vi "ADC_DAC_Trigger.vi"() -> ()   [LabVIEW 2018]
doc: "The DtAinContinuous example demonstrates how to continuously acquire data from an analog input channel. This example runs continuously until either the Stop button is pressed or an error occurs."
uses:
  <userlib>/LV-Link3/PolySubVIs/DtCreateAinChan.vi
  <userlib>/LV-Link3/PolySubVIs/DtOLWriteMultiple2D.vi
  <userlib>/LV-Link3/PolySubVIs/DtOLTimingSetInput.vi
  <vilib>/Waveform/WDTFileIO.llb/Export Waveform To Spreadsheet File.vi
  <vilib>/Analysis/baseanly.llb/Mean (DBL).vi
  <vilib>/Analysis/NI_AALBase.lvlib
  <vilib>/measure/mamon.llb/Trigger Detection for 1 Channel.vi
  <vilib>/measure/NI_MAPro.lvlib
  <userlib>/LV-Link3/PolySubVIs/DtCreateAoutChan.vi
panel:
  in  "Tab Control":T1(tab)
  in  "Device":string(combo)="DT9816-S(00)"
  in  "Device 2":string(combo)="DT9854(00)"
  in  "ADC Channels":string="0, 1, 2, 3, 4"
  in  "Sample Rate":u32=10000
  in  "Samples Per Channel":i32=1000
  in  "Sync Mode":i32(ring) items=["None", "Master", "Slave"]
  in  "Start Button":bool
  in  "Stop Button":bool
  in  "DAC Channels":string="0, 1, 2, 3, 4"
  in  "?":bool
  in  "Trigger Channel":i8 min=0 max=5
  in  "location mode":u16(ring) items=["Index", "Time"]
  in  "trigger slope":u16(ring)=1 items=["Falling Edge", "Rising Edge"]
  in  "DAC Channel 0":dbl=0.22199999999999995 min=0.0 max=1.125 step=0.01
  in  "DAC Channel 1":dbl=0.5200000000000001 min=0.0 max=1.125 step=0.01
  in  "DAC Channel 2":dbl=0.42000000000000015 min=0.0 max=1.125 step=0.01
  in  "DAC Channel 3":dbl=0.41000000000000014 min=0.0 max=1.125 step=0.01
  in  "DAC Channel 4":dbl=0.5200000000000001 min=0.0 max=1.125 step=0.01
  out "Signal from two channel":dbl[][](graph)
  out "Signal from two channel":dbl[][](graph)
  out "Waveform Chart":dbl(graph)
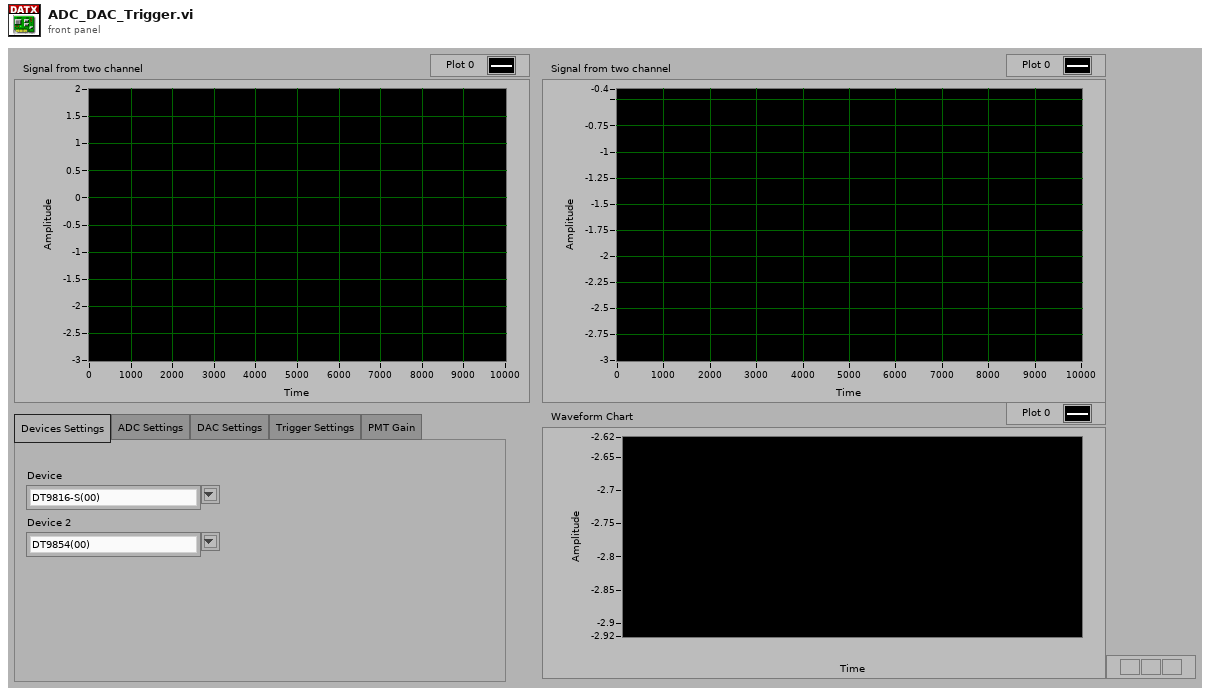
[diagram p1: front panel]
types:
  T1 = enum32{"Devices Settings", "ADC Settings", "DAC Settings", "Trigger Settings", "PMT Gain"}
  T2 = enum8{"Enabled", "Disabled", "Disabled and Grayed Out"}
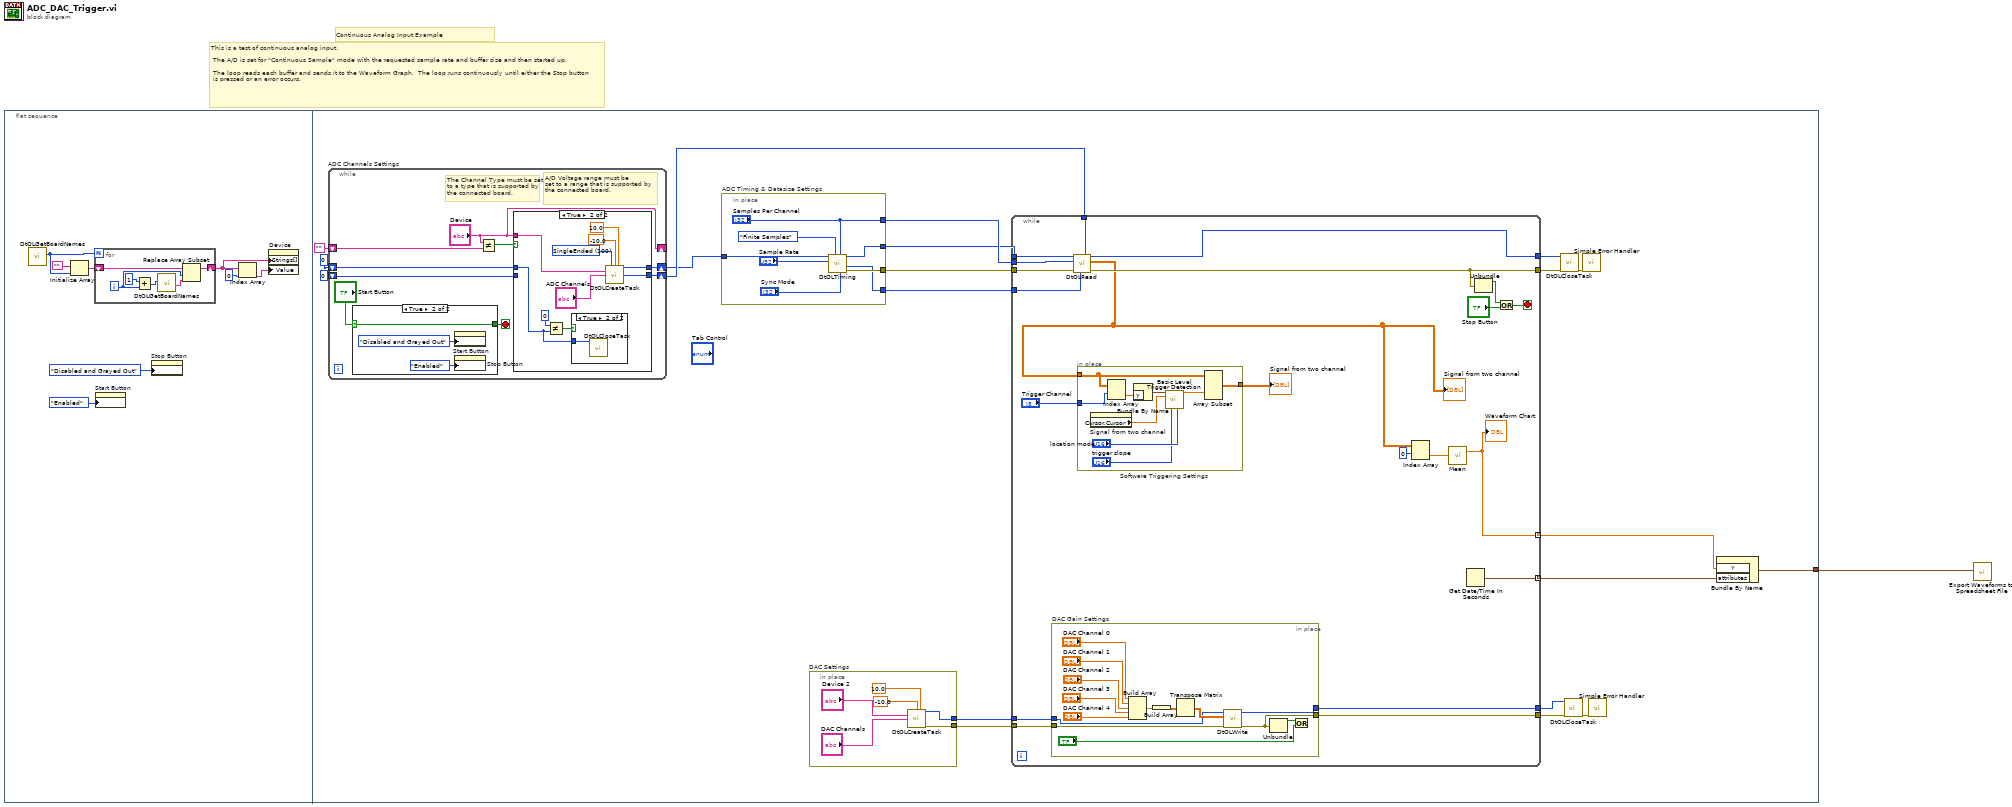
[diagram p0: block diagram]
diagram:
  # "Continuous Analog Input Example"
  # "This is a test of continuous analog input. \n\n The A/D is set for \"Continuous Sample\" mode with the requested sample rate and buffer size and then started up.\n\n The loop reads each buffer and sends it to the Waveform Graph.  The loop runs continuously until either the Stop button\n is pressed or an error occurs."
  n1 = flat-sequence {
    tunnel: [w23] -> w1
    frame #0 {
      n2 = call <userlib>:"DtOLGetBoardNames.vi"() -> ("Number of boards"=w9:u32)  [unwired: 9 in, 2 out]
      n3 = Initialize Array "Initialize Array"("", w9) -> (w7:string[])
      n4 = for {
        N: w9 -> [_]
        shift-right: [w12] -> w4
        shift-left: w7 -> [w13]
        i -> [w11]
        n5 = Add(x=1, y=w11) -> (x+y=w15:i32)
        n6 = call <userlib>:"DtOLGetBoardNames.vi"("Select Board"=w15) -> ("Board Name"=w10:string)  [unwired: 8 in, 2 out]
        n7 = Replace Array Subset(array=w13, new element=w10, index=w11) -> (w12:string[])
      }
      n8 = property on="Start Button" class="Bool"("DisabledEnum"=T2."Enabled" ("Disabled")) -> ()  [unwired: 2 in, 2 out]
      n9 = property on="Stop Button" class="Bool"("DisabledEnum"=T2."Disabled and Grayed Out" ("Disabled")) -> ()  [unwired: 2 in, 2 out]
      n10 = Index Array(array=w4, index=0) -> (element=w5:string)
      n11 = property on="Device" class="CmbBox"("Strings[]"=w4, "Value"=w5) -> ()  [unwired: 2 in, 2 out]
    }
    frame #1 {
      n12 = while "ADC Channels Settings" {
        shift-right: ["Device"] -> _
        shift-left: "" -> [w57]
        shift-right: [w54] -> w19
        shift-left: 0 ("Task out") -> [w55]
        shift-right: [w52] -> w29
        shift-left: u32 0 ("Actual Number of Channels") -> [w51]
        stop <- w53 stop-if-true
        # "The Channel Type must be set\nto a type that is supported by \nthe connected board."
        # "A/D Voltage range must be\nset to a range that is supported by \nthe connected board."
        n13 = case shown="True" "Start Button" {
          selector: "Start Button" -> [w59 w62]
          tunnel: [w59 w62] -> w53
          frame False {
          }
          frame True {
            n14 = property on="Start Button" class="Bool"("DisabledEnum"=T2."Disabled and Grayed Out" ("Disabled")) -> ()  [unwired: 2 in, 2 out]
            n15 = property on="Stop Button" class="Bool"("DisabledEnum"=T2."Enabled" ("Disabled")) -> ()  [unwired: 2 in, 2 out]
          }
        }
        n16 = Not Equal?(x="Device", y=w57) -> (x != y?=w58:bool)
        n17 = case shown="True" w58 {
          tunnel: "Device" -> [_ w71]
          tunnel: [w64 w70] -> w54
          tunnel: w55 -> [w64 w67]
          tunnel: [w63 w65] -> w52
          tunnel: w51 -> [w63 _]
          frame False {
          }
          frame True {
            w72 = 100 items=["SingleEnded"=100, "Differential"=101] ("Channel Type")
            n18 = Not Equal?(x=0, y=w67) -> (x != y?=w68:bool)
            n19 = case shown="True" w68 {
              tunnel: w67 -> [_ w75]
              frame False {
              }
              frame True {
                n20 = call <userlib>:"DtOLCloseTask.vi"("Task in"=w75) -> ()  [unwired: 10 in, 1 out]
              }
            }
            n21 = call-poly <userlib>:"DtOLCreateTask.vi"("Channel Type"=w72, "Range Min"=-10.0, "Range Max"=10.0, "Board Name"=w71, "Channel"="ADC Channels") -> ("Task out"=w70:i32, "Actual Number of Channels"=w65:u32)  [unwired: 8 in, 1 out]
          }
        }
      }
      n22 = in-place "ADC Timing & Datasize Settings" {
        in-place-border: ["Samples Per Channel"] -> w20
        in-place-border: w19 -> [w39]
        in-place-border: [w38] -> w18
        in-place-border: [w37] -> w17
        in-place-border: [w36] -> w16
        n23 = call-poly <userlib>:"DtOLTiming.vi"("Sync Mode"="Sync Mode", "Samples Per Channel"="Samples Per Channel", "Sample Mode"=enum16{"Finite Samples", "Continuous Samples"}."Finite Samples", "Sample Freq (Hz)"="Sample Rate", "Task in"=w39) -> ("error out"=w38:errorcluster, "Buffer Size"=w37:u32, "Task out"=w36:i32)  [unwired: 3 in, 1 out]
      }
      n24 = in-place "DAC Settings" {
        in-place-border: [w45] -> w22
        in-place-border: [w44] -> w21
        n25 = call-poly <userlib>:"DtOLCreateTask.vi"("Range Min"=-10.0, "Range Max"=10.0, "Board Name"="Device 2", "Channel"="DAC Channels") -> ("Task out"=w45:i32, "error out"=w44:errorcluster)  [unwired: 9 in, 1 out]
      }
      n26 = while {
        tunnel: w18 -> [w85]
        tunnel: [w96] -> w34
        tunnel: [w95] -> w35
        tunnel: w16 -> [w86]
        tunnel: w29 -> [w91]
        tunnel: w17 -> [w84]
        tunnel: [w90] -> w27
        tunnel: [w89] -> w26
        tunnel: w22 -> [w88]
        tunnel: w21 -> [w87]
        tunnel: [w81] -> w25 mode=indexing
        tunnel: [w80] -> w24 mode=indexing
        tunnel: w20 -> [w79]
        stop <- w92 stop-if-true
        n27 = in-place "DAC Gain Settings" {
          in-place-border: [w110] -> w90
          in-place-border: [w109] -> w89
          in-place-border: w88 -> [w108]
          in-place-border: w87 -> [w107]
          n28 = Build Array("DAC Channel 0", "DAC Channel 1", "DAC Channel 2", "DAC Channel 3", "DAC Channel 4") -> (w118:dbl[])
          n29 = Build Array(w118) -> (w106:dbl[][])
          n30 = Transpose Matrix(1:w106) -> (0:w119:dbl[][])
          n31 = call-poly <userlib>:"DtOLWrite.vi"("error in (no error)"=w107, "Data in"=w119, "Task in"=w108) -> ("error out"=w109:errorcluster, "Task out"=w110:i32)  [unwired: 6 in, 1 out]
          n32 = Unbundle(w109) -> ("status"=w111:bool)  [unwired: 2 out]
          n33 = Or(x=w111, y="?") -> ()  [unwired: 1 out]
        }
        n34 = call-poly <userlib>:"DtOLRead.vi"("Number Chan to Read"=w91, "Buffer size"=w84, "error in (no error)"=w85, "Samples Per Channel"=w79, "Task in"=w86) -> ("error out"=w95:errorcluster, "2D Data out"=w77:dbl[][], "Task out"=w96:i32)  [unwired: 2 in, 2 out]
        "Signal from two channel" <- w77
        n35 = in-place "Software Triggering Settings" {
          in-place-border: [w99] -> w78
          in-place-border: w77 -> [w98]
          in-place-border: "Trigger Channel" -> [w97]
          n36 = property on="Signal from two channel" class="WFGraph (strict)"() -> ("Cursor.Cursor Y"=w101:dbl)  [unwired: 2 in, 2 out]
          n37 = Index Array(array=w98, index (row)=w97) -> (element=w105:dbl[])  [unwired: 1 in]
          n38 = Bundle By Name("Y"=w105) -> (w104:waveform(dbl))  [unwired: 1 in]
          n39 = call-poly <vilib>:"Basic Level Trigger Detection.vi"("signal in"=w104, "level"=w101, "location mode"="location mode", "trigger slope"="trigger slope") -> ("trigger location"=w100:dbl)  [unwired: 9 in, 2 out]
          n40 = Array Subset(array=w98, index (col)=w100) -> (w99:dbl[][])  [unwired: 3 in]
        }
        "Signal from two channel" <- w78
        n41 = Index Array "Index Array"(array=w77, index (row)=0) -> (element=w82:dbl[])  [unwired: 1 in]
        n42 = call-poly <vilib>:"Mean.vi"("X"=w82) -> ("mean"=w81:dbl)  [unwired: 1 out]
        "Waveform Chart" <- w81
        n43 = Get Date/Time In Seconds() -> (seconds since 1Jan1904=w80:timestamp)
        n44 = Unbundle(w95) -> ("status"=w94:bool)  [unwired: 2 out]
        n45 = Or(x=w94, y="Stop Button") -> (x .or. y?=w92:bool)
      }
      n46 = call <userlib>:"DtOLCloseTask.vi"("Error in"=w35, "Task in"=w34) -> ("Error Out"=w33:errorcluster)  [unwired: 9 in]
      n47 = call <userlib>:"DtOLCloseTask.vi"("Error in"=w26, "Task in"=w27) -> ("Error Out"=w28:errorcluster)  [unwired: 9 in]
      n48 = call <vilib>:"Simple Error Handler.vi"("error in (no error)"=w33) -> ()  [unwired: 4 in, 5 out]
      n49 = call <vilib>:"Simple Error Handler.vi"("error in (no error)"=w28) -> ()  [unwired: 4 in, 5 out]
      n50 = Bundle By Name("Y"=w25, "attributes"=w24) -> (w23:waveform(dbl))  [unwired: 1 in]
    }
  }
  n51 = call-poly <vilib>:"Export Waveforms to Spreadsheet File.vi"("waveform"=w1) -> ()  [unwired: 9 in, 2 out]
